vi "View Edit Parameters.vi"(1 "Subject Parameters In":T1 {"Subject" items=["Subject 0", "Subject 1", "Subject 2", "Subject 3", "Subject 4", "Subject 5", "Subject 6", "Subject 7", "Subject 8", "Subject 9", "Subject 10", "Subject 11", "Subject 12", "Subject 13", "Subject 14", "Subject 15", "Subject 16", "Subject 17", "Subject 18", "Subject 19", "Subject 20", "Subject 21", "Subject 22", "Subject 23", "Subject 24", "Subject 25", "Subject 26", "Subject 27", "Subject 28", "Subject 29", "Subject 30", "Subject 31", "Subject 32", "Subject 33", "Subject 34", "Subject 35", "Subject 36", "Subject 37", "Subject 38", "Subject 39", "Subject 40"]}) -> (0 "Subject Parameters Out":T1 {"Subject" items=["Subject 0", "Subject 1", "Subject 2", "Subject 3", "Subject 4", "Subject 5", "Subject 6", "Subject 7", "Subject 8", "Subject 9", "Subject 10", "Subject 11", "Subject 12", "Subject 13", "Subject 14", "Subject 15", "Subject 16", "Subject 17", "Subject 18", "Subject 19", "Subject 20", "Subject 21", "Subject 22", "Subject 23", "Subject 24", "Subject 25", "Subject 26", "Subject 27", "Subject 28", "Subject 29", "Subject 30", "Subject 31", "Subject 32", "Subject 33", "Subject 34", "Subject 35", "Subject 36", "Subject 37", "Subject 38", "Subject 39", "Subject 40"]})   [LabVIEW 2019]
uses:
  Controls/Subject Params.ctl
  Controls/Subject.ctl
  Controls/GPD Side Parameters.ctl
  Controls/Type Defs/Stim Parameters.ctl
  Controls/Stim off-half-ful.ctl
panel:
  in  "Done":bool
  in  "Subject Parameters":T1 {"Subject" items=["Subject 0", "Subject 1", "Subject 2", "Subject 3", "Subject 4", "Subject 5", "Subject 6", "Subject 7", "Subject 8", "Subject 9", "Subject 10", "Subject 11", "Subject 12", "Subject 13", "Subject 14", "Subject 15", "Subject 16", "Subject 17", "Subject 18", "Subject 19", "Subject 20", "Subject 21", "Subject 22", "Subject 23", "Subject 24", "Subject 25", "Subject 26", "Subject 27", "Subject 28", "Subject 29", "Subject 30", "Subject 31", "Subject 32", "Subject 33", "Subject 34", "Subject 35", "Subject 36", "Subject 37", "Subject 38", "Subject 39", "Subject 40"]}
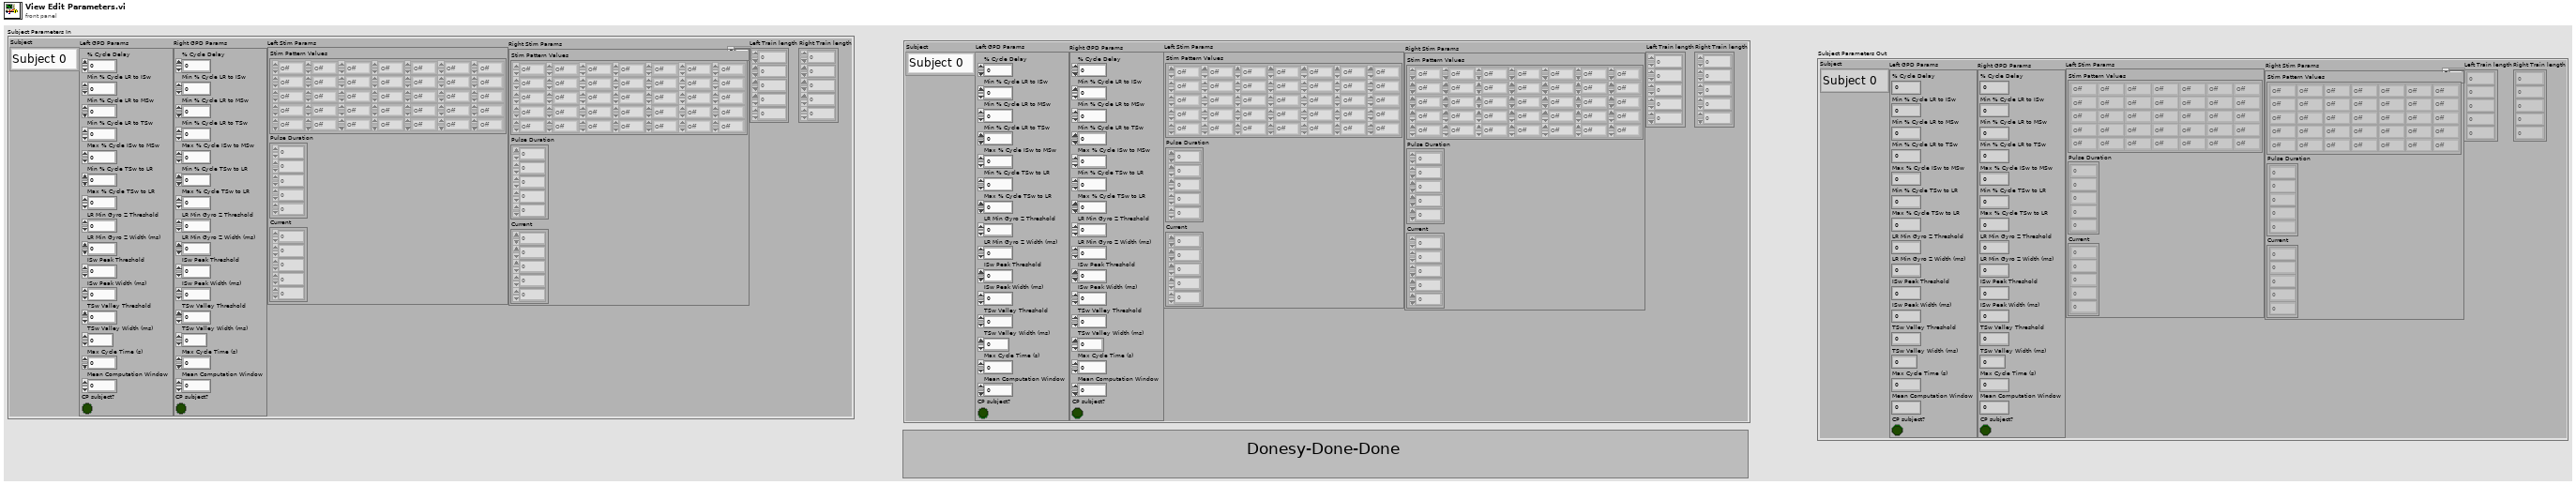
[diagram p1: front panel]
types:
  T1 = typedef "Subject Params.ctl" = cluster{"Subject":T2, "Left GPD Params":T3, "Right GPD Params":T3, "Left Stim Params":T4, "Right Stim Params":T4, "Left Train length":i64[], "Right Train length":i64[]}
  T2 = typedef "Subject.ctl" = u16
  T3 = typedef "GPD Side Parameters.ctl" = cluster{"% Cycle Delay":dbl, "Min % Cycle LR to ISw ":dbl, "Min % Cycle LR to MSw":dbl, "Min % Cycle LR to TSw":dbl, "Max % Cycle ISw to MSw":dbl, "Min % Cycle TSw to LR":dbl, "Max % Cycle TSw to LR":dbl, "LR Min Gyro Z Threshold":dbl, "LR Min Gyro Z Width":dbl, "ISw Peak Threshold":dbl, "ISw Peak Width":dbl, "TSw Valley Threshold":dbl, "TSw Valley Width (ms)":dbl, "Max Cycle Time (s)":dbl, "Mean Computation Window":dbl, "CP subject?":bool}
  T4 = typedef "Stim Parameters.ctl" = cluster{"Stim Pattern Values":T5[][], "Pulse Duration":i64[], "Current":i64[]}
  T5 = typedef "Stim off-half-ful.ctl" = enum16{"Off", "Half", "Full"}
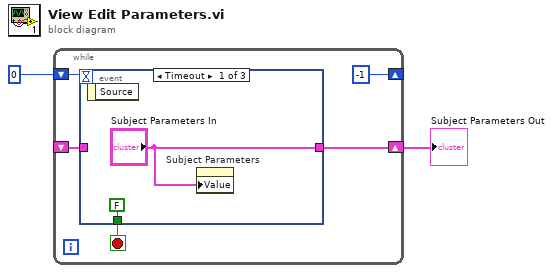
[diagram p0: block diagram]
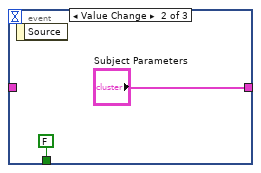
[diagram p2: hidden frame]
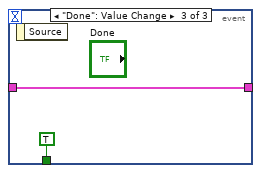
[diagram p3: hidden frame]
diagram:
  n1 = while {
    shift-right: [-1] -> _
    shift-left: 0 -> [w7]
    shift-right: [w4] -> w1
    shift-left: _ -> [w3]
    stop <- w5 stop-if-true
    n2 = event shown="[0] Timeout" {
      selector: _ -> [_ _ _]
      dyn-events: _ -> [_ _ _]
      timeout: w7 -> [_ _ _]
      tunnel: [FALSE FALSE TRUE] -> w5
      tunnel: ["Subject Parameters In" "Subject Parameters" w12] -> w4
      tunnel: w3 -> [_ _ w12]
      event Timeout {
        n3 = event-data() -> ()  [unwired: 1 in, 1 out]
        n4 = property on="Subject Parameters" class="Clust (strict)"("Value"="Subject Parameters In") -> ()  [unwired: 2 in, 2 out]
      }
      event Value Change {
        n5 = event-data() -> ()  [unwired: 1 in, 1 out]
      }
      event "Done": Value Change {
        n6 = event-data() -> ()  [unwired: 1 in, 1 out]
      }
    }
  }
  "Subject Parameters Out" <- w1
